vi "Create.vi"(8 "error in (no error)":errorcluster, 11 "Config Folder":path=path "C:/Users/dustindam/Desktop/gantry/Config") -> (0 "error out":errorcluster, 3 "WorkTable Class out":refnum<class "WorkTable Class.lvclass">)   [LabVIEW 2011, in "WorkTable Class.lvclass"]
uses:
  WorkTable Class.lvclass
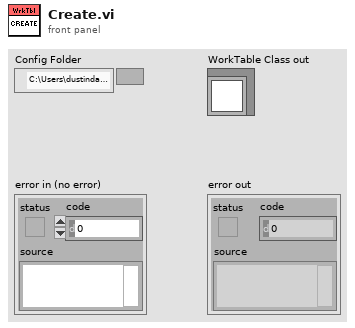
[diagram p1: front panel]
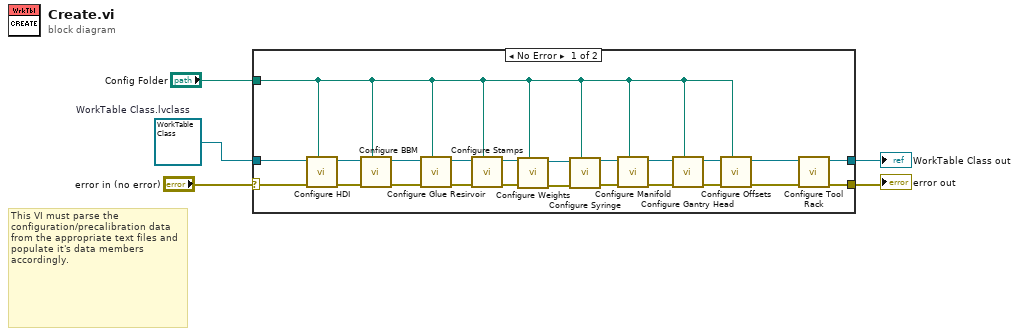
[diagram p0: block diagram]
diagram:
  w5 = refnum<class "WorkTable Class.lvclass"> refnum  # WorkTable Class.lvclass
  # "This VI must parse the configuration/precalibration data from the appropriate text files and populate it's data members accordingly."
  n1 = case shown="No Error" "error in (no error)" {
    selector: "error in (no error)" -> [w23 w30]
    tunnel: w5 -> [w28 w29]
    tunnel: [w16 w29] -> w4
    tunnel: [w15 w30] -> w3
    tunnel: "Config Folder" -> [w8 _]
    frame No Error {
      n2 = call "Configure HDI.vi"("Config Folder"=w8, "error in (no error)"=w23, "WorkTable Class in"=w28) -> ("error out"=w26:errorcluster, "WorkTable Class out"=w27:refnum<class "WorkTable Class.lvclass">)  [unwired: 7 in]
      n3 = call "Configure BBM.vi"("Config Folder"=w8, "error in (no error)"=w26, "WorkTable Class in"=w27) -> ("error out"=w24:errorcluster, "WorkTable Class out"=w25:refnum<class "WorkTable Class.lvclass">)  [unwired: 7 in]
      n4 = call "Configure Glue Resirvoir.vi"("Config Folder"=w8, "error in (no error)"=w24, "WorkTable Class in"=w25) -> ("error out"=w21:errorcluster, "WorkTable Class out"=w22:refnum<class "WorkTable Class.lvclass">)  [unwired: 7 in]
      n5 = call "Configure Stamps.vi"("Config Folder"=w8, "error in (no error)"=w21, "WorkTable Class in"=w22) -> ("error out"=w19:errorcluster, "WorkTable Class out"=w20:refnum<class "WorkTable Class.lvclass">)  [unwired: 7 in]
      n6 = call "Configure Weights.vi"("Config Folder"=w8, "error in (no error)"=w19, "WorkTable Class in"=w20) -> ("error out"=w17:errorcluster, "WorkTable Class out"=w18:refnum<class "WorkTable Class.lvclass">)  [unwired: 7 in]
      n7 = call "Configure Syringe.vi"("Config Folder"=w8, "error in (no error)"=w17, "WorkTable Class in"=w18) -> ("error out"=w13:errorcluster, "WorkTable Class out"=w14:refnum<class "WorkTable Class.lvclass">)  [unwired: 7 in]
      n8 = call-dynamic "Configure Manifold.vi"("Config Folder"=w8, "error in (no error)"=w13, "WorkTable Class in"=w14) -> ("error out"=w11:errorcluster, "WorkTable Class out"=w12:refnum<class "WorkTable Class.lvclass">)  [unwired: 7 in]
      n9 = call-dynamic "Configure Gantry Head.vi"("Config Folder"=w8, "error in (no error)"=w11, "WorkTable Class in"=w12) -> ("error out"=w9:errorcluster, "WorkTable Class out"=w10:refnum<class "WorkTable Class.lvclass">)  [unwired: 7 in]
      n10 = call-dynamic "Configure Offsets.vi"("Config Folder"=w8, "error in (no error)"=w9, "WorkTable Class in"=w10) -> ("error out"=w6:errorcluster, "WorkTable Class out"=w7:refnum<class "WorkTable Class.lvclass">)  [unwired: 7 in]
      n11 = call "Configure Tool Rack.vi"("error in (no error)"=w6, "WorkTable Class in"=w7) -> ("error out"=w15:errorcluster, "WorkTable Class out"=w16:refnum<class "WorkTable Class.lvclass">)  [unwired: 8 in]
    }
    frame Error {
    }
  }
  "error out" <- w3
  "WorkTable Class out" <- w4
